vi ".NET Datatype Information to G Data Type Information.vi"(8 "error in (no error)":errorcluster, 9 ".NET Data Type Information":refnum<k24>, 11 "TwinCAT ADS in":refnum<class "TwinCAT ADS.lvclass">) -> (0 "error out":errorcluster, 2 "Data Type Information":T1 {"Category" items=["Unknown, None"=0, "Primitive"=1, "Alias"=2, "Enum"=3, "Array"=4, "Struct"=5, "FunctionBlock"=6, "Program"=7, "Function"=8, "SubRange"=9, "String"=10, "Bitset"=12, "Pointer"=13, "Union"=14, "Reference"=15, "Interface"=16]; "Type ID" items=["ADST_VOID"=0, "ADST_INT16"=2, "ADST_INT32"=3, "ADST_REAL32"=4, "ADST_REAL64"=5, "ADST_INT8"=16, "ADST_UINT8"=17, "ADST_UINT16"=18, "ADST_UINT32"=19, "ADST_INT64"=20, "ADST_UINT64"=21, "ADST_STRING"=30, "ADST_WSTRING"=31, "ADST_REAL80"=32, "ADST_BIT"=33, "ADST_MAXTYPES"=34, "ADST_BIGTYPE"=65]}, 3 "TwinCAT ADS out":refnum<class "TwinCAT ADS.lvclass">)   [LabVIEW 2018, in "TwinCAT ADS.lvclass"]
uses:
  TwinCAT ADS.lvclass
  TwinCAT.Ads
  Controls/Datatype Information.ctl
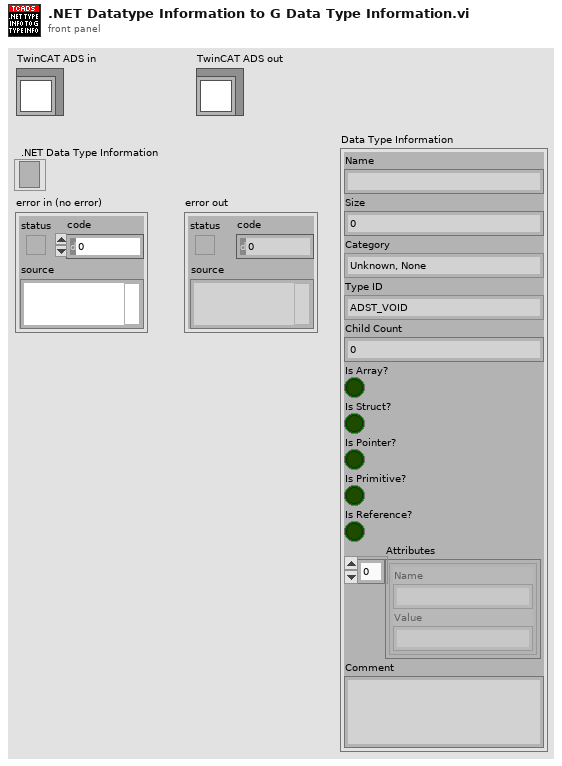
[diagram p1: front panel]
types:
  T1 = typedef "TwinCAT ADS.lvclass/Datatype Information.ctl" = cluster{"Name":string, "Size":i32, "Category":i32, "Type ID":i32, "Child Count":i32, "Is Array?":bool, "Is Struct?":bool, "Is Pointer?":bool, "Is Primitive?":bool, "Is Reference?":bool, "Attributes":cluster{"Name":string, "Value":string}[], "Comment":string}
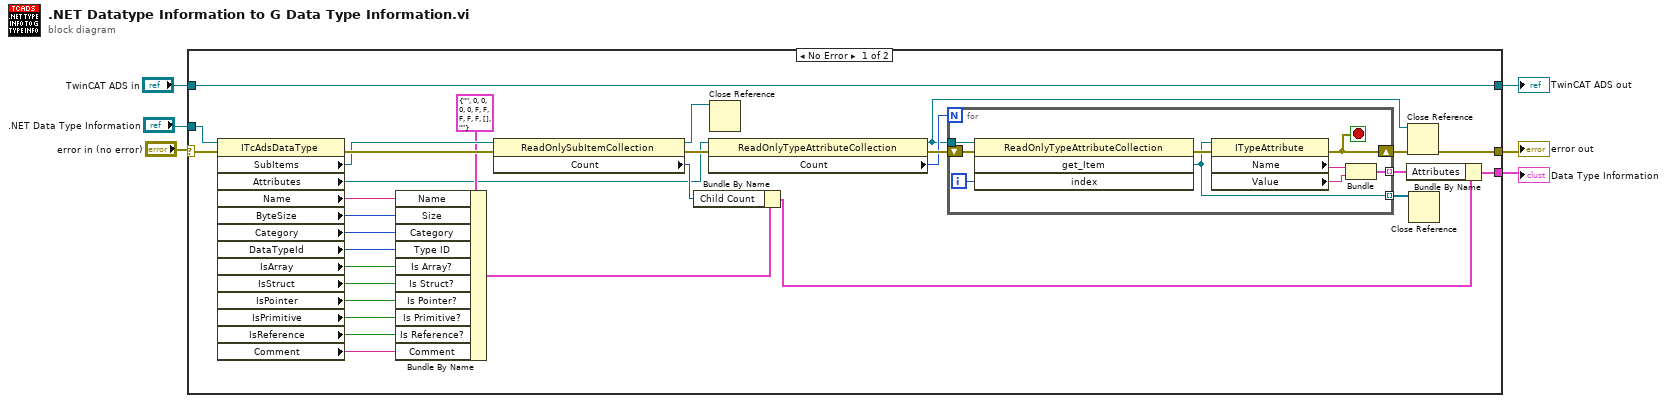
[diagram p0: block diagram]
diagram:
  n1 = case shown="No Error" "error in (no error)" {
    selector: "error in (no error)" -> [w35 w47]
    tunnel: [w7 w47] -> w5
    tunnel: [w36 w46] -> w3
    tunnel: "TwinCAT ADS in" -> [w36 w46]
    tunnel: ".NET Data Type Information" -> [w34 _]
    tunnel: [w21 _] -> w1
    frame No Error {
      n2 = property class="ITcAdsDataType"(reference=w34, error in=w35) -> (error out=w19:errorcluster, "SubItems"=w15:refnum<k24>, "Attributes"=w12:refnum<k24>, "Name"=w33:string, "ByteSize"=w32:i32, "Category"=w31:i32, "DataTypeId"=w30:i32, "IsArray"=w20:bool, "IsStruct"=w29:bool, "IsPointer"=w28:bool, "IsPrimitive"=w27:bool, "IsReference"=w26:bool, "Comment"=w25:string)  [unwired: 1 out]
      n3 = Bundle By Name(cluster=T1 {"Name"="", "Size"=0, "Category"=0, "Type ID"=0, "Child Count"=0, "Is Array?"=FALSE, "Is Struct?"=FALSE, "Is Pointer?"=FALSE, "Is Primitive?"=FALSE, "Is Reference?"=FALSE, "Attributes"=[], "Comment"=""} ("Data Type Information"), "Name"=w33, "Size"=w32, "Category"=w31, "Type ID"=w30, "Is Array?"=w20, "Is Struct?"=w29, "Is Pointer?"=w28, "Is Primitive?"=w27, "Is Reference?"=w26, "Comment"=w25) -> (w18:T1)
      n4 = property class="ReadOnlySubItemCollection"(reference=w15, error in=w19) -> (reference out=w11:refnum<k24>, error out=w13:errorcluster, "Count"=w17:i32)
      n5 = Bundle By Name(cluster=w18, "Child Count"=w17) -> (w16:T1)
      n6 = property class="ReadOnlyTypeAttributeCollection"(reference=w12, error in=w13) -> (reference out=w9:refnum<k24>, error out=w24:errorcluster, "Count"=w23:i32)
      n7 = Close Reference(reference=w11) -> ()  [unwired: 1 in, 1 out]
      n8 = for {
        N: w23 -> [_]
        tunnel: w9 -> [w45]
        tunnel: [w40] -> w22 mode=indexing
        shift-right: [w38] -> w8
        shift-left: w24 -> [w39]
        tunnel: [w37] -> w10 mode=indexing
        i -> [w44]
        stop <- w38 stop-if-true
        n9 = invoke class="ReadOnlyTypeAttributeCollection" method="get_Item"(reference=w45, error in=w39, "index"=w44) -> (error out=w43:errorcluster, "get_Item"=w37:refnum<k24>)  [unwired: 1 in, 2 out]
        n10 = property class="ITypeAttribute"(reference=w37, error in=w43) -> (error out=w38:errorcluster, "Name"=w42:string, "Value"=w41:string)  [unwired: 1 out]
        n11 = Bundle("Name"=w42, "Value"=w41) -> (w40:cluster{"Name":string, "Value":string})  [unwired: 1 in]
      }
      n12 = Bundle By Name(cluster=w16, "Attributes"=w22) -> (w21:T1)
      n13 = Close Reference(reference=w9, error in (no error)=w8) -> (error out=w7:errorcluster)
      n14 = Close Reference(reference=w10) -> ()  [unwired: 1 in, 1 out]
    }
    frame Error {
    }
  }
  "error out" <- w5
  "TwinCAT ADS out" <- w3
  "Data Type Information" <- w1
